vi "WaveformTimeShift.vi"(0 "Waveform In":waveform(dbl), 1 "Time Shift":dbl format="%.3g") -> (2 "Waveform Out":waveform(dbl))   [LabVIEW 2009]
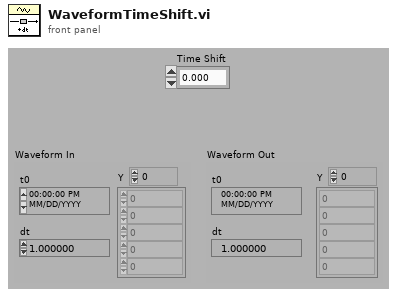
[diagram p1: front panel]
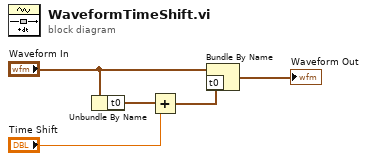
[diagram p0: block diagram]
diagram:
  n1 = Unbundle By Name("Waveform In") -> ("t0"=w3:timestamp)
  n2 = Add(x=w3, y="Time Shift") -> (x+y=w2:timestamp)
  n3 = Bundle By Name(cluster="Waveform In", "t0"=w2) -> (→"Waveform Out":waveform(dbl))
